vi "Read.vi"(8 "error in (no error)":errorcluster, 9 "Variant":variant, 11 "Ethernet in":refnum<class "TCP.lvclass">) -> (0 "error out":errorcluster, 2 "String":string, 3 "Ethernet out":refnum<class "TCP.lvclass">)   [LabVIEW 2019, in "Localhost Protocols.lvlib" / "TCP.lvclass"]
uses:
  TCP.lvclass
  Protocol Parent/Methods/Read Parameter.ctl
  TCP.lvclass/TCP.ctl
  Data Access/Read TCP Ref.vi
  Data Access/Write TCP Ref.vi
  <vilib>/Utility/error.llb/Clear Errors.vi
  Protocol Parent/Protocol Parent.lvclass
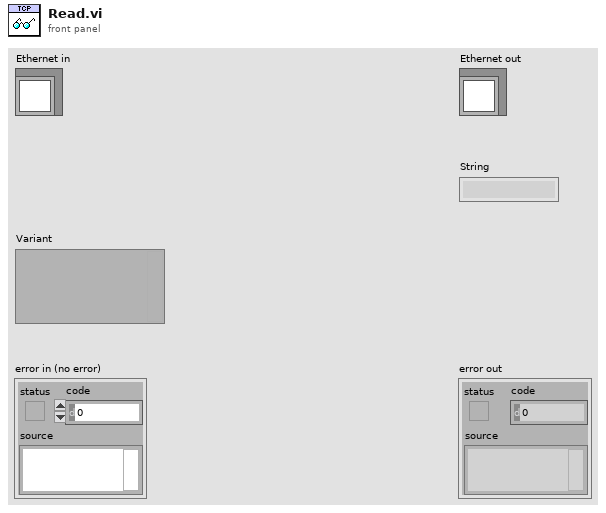
[diagram p1: front panel]
types:
  T1 = typedef "Localhost Protocols.lvlib/Protocol Parent.lvclass/Read Parameter.ctl" = cluster{"Wait Type":enum16{"Byte Count", "Wait sec"}, "Wait Value":dbl}
  T2 = enum16{"Standard", "Buffered", "CRLF", "Immediate"}
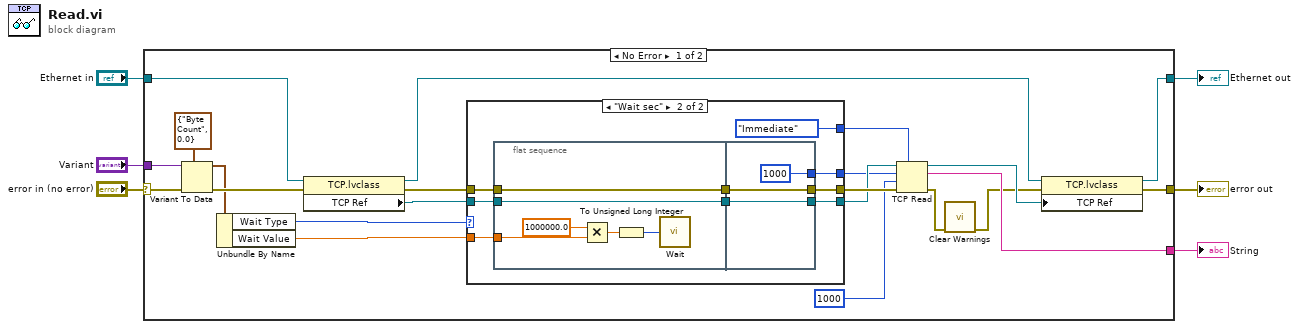
[diagram p0: block diagram]
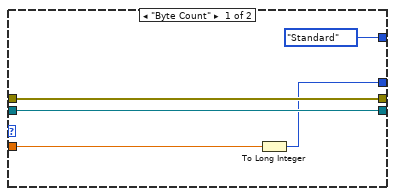
[diagram p2: hidden frame]
diagram:
  n1 = case shown="No Error" "error in (no error)" {
    selector: "error in (no error)" -> [w23 w53]
    tunnel: "Ethernet in" -> [w28 w52]
    tunnel: [w26 w53] -> w3
    tunnel: [w24 w52] -> w2
    tunnel: "Variant" -> [w21 _]
    tunnel: [w12 _] -> w1
    frame No Error {
      n2 = Variant To Data(error in=w23, type=T1 {"Wait Type"=enum."Byte Count", "Wait Value"=0.0} ("Read Parameter"), Variant=w21) -> (data=w20:T1, error out=w22:errorcluster)
      n3 = Unbundle By Name(w20) -> ("Wait Type"=w14:enum16{"Byte Count", "Wait sec"}, "Wait Value"=w13:dbl)
      n4 = property class="TCP.lvclass"(reference=w28, error in=w22) -> (reference out=w25:refnum<class "TCP.lvclass">, error out=w19:errorcluster, "TCP Ref"=w18:refnum<k5>)
      n5 = case shown="\"Wait sec\"" w14 {
        tunnel: w19 -> [w33 w42]
        tunnel: w18 -> [w31 w41]
        tunnel: [w33 w40] -> w17
        tunnel: [w31 w39] -> w16
        tunnel: [w29 w35] -> w15
        tunnel: w13 -> [w32 w36]
        tunnel: [T2."Standard" ("mode (standard)") T2."Immediate" ("mode (standard)")] -> w10
        frame "Byte Count" {
          n6 = To Long Integer(number=w32) -> (32bit integer=w29:i32)
        }
        frame "Wait sec" {
          n7 = flat-sequence {
            tunnel: w41 -> [w47]
            tunnel: w42 -> [w48]
            tunnel: [w48] -> w38
            tunnel: [w47] -> w37
            tunnel: w36 -> [w46]
            tunnel: [w51] -> w40
            tunnel: [w50] -> w39
            tunnel: w38 -> [w51]
            tunnel: w37 -> [w50]
            tunnel: [1000 ("Wait Value")] -> w35
            frame #0 {
              n8 = Multiply(x=1000000.0, y=w46) -> (x*y=w45:dbl)
              n9 = To Unsigned Long Integer(number=w45) -> (unsigned 32bit integer=w43:u32)
              n10 = call "Wait"("Count(uSec)"=w43) -> ()  [unwired: 1 out]
            }
            frame #1 {
            }
          }
        }
      }
      n11 = TCP Read(connection ID=w16, bytes to read=w15, error in (no error)=w17, 7:w10, 9:1000 ("timeout ms (25000)")) -> (connection ID out=w27:refnum<k5>, data out=w12:string, error out=w8:errorcluster)
      n12 = call "Clear Warnings.vi"("error in (no error)"=w8) -> ("error out"=w7:errorcluster)  [unwired: 10 in]
      n13 = property class="TCP.lvclass"(reference=w25, error in=w7, "TCP Ref"=w27) -> (reference out=w24:refnum<class "TCP.lvclass">, error out=w26:errorcluster)
    }
    frame Error {
    }
  }
  "error out" <- w3
  "Ethernet out" <- w2
  "String" <- w1
